vi "cCRDS Server.vi"(11 "cCRDS":refnum<class "cCRDS.lvclass">) -> ()   [LabVIEW 2015]
uses:
  cCRDS.lvclass
  Reusable/Instrument/state.ctl
  Reusable/CRDS/Main/CRDS.lvclass/CRDS.ctl
  Reusable/CRDS/Main/Read CRD RD Data Obs.vi
  Reusable/CRDS/Main/Write CRD RD Data Obs.vi
  Reusable/File IO/Class/File Observer.lvclass
  Reusable/Instrument/Instrument.lvclass
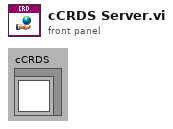
[diagram p1: front panel]
types:
  T1 = typedef "Instrument.lvclass/state.ctl" = enum8{"Configure", "Acquire", "Wait", "Quit", "Handle Error", "NOOP"}
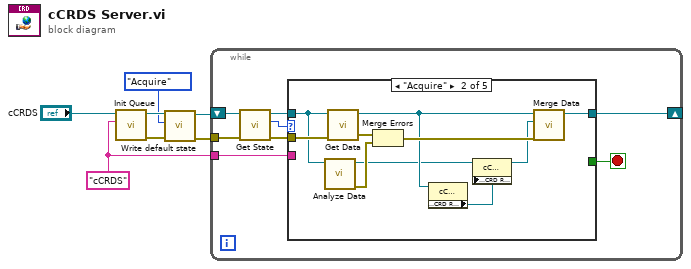
[diagram p0: block diagram]
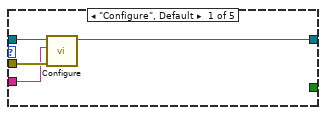
[diagram p2: hidden frame]
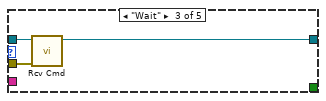
[diagram p3: hidden frame]
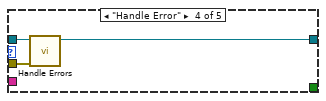
[diagram p4: hidden frame]
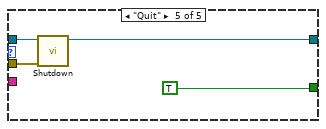
[diagram p5: hidden frame]
diagram:
  w4 = "cCRDS" ("queue_name")
  n1 = call "Init Queue.vi"("queue_name"=w4, "Instrument in"="cCRDS") -> ("error out"=w6:errorcluster, "Instrument out"=w7:refnum<class "cCRDS.lvclass">)  [unwired: 8 in]
  n2 = call "Write default state.vi"("error in (no error)"=w6, "instr state"=state."Acquire", "Instrument in"=w7) -> ("error out"=w1:errorcluster, "Instrument out"=w2:refnum<class "cCRDS.lvclass">)  [unwired: 7 in]
  n3 = while "Acquisition" {
    tunnel: w1 -> [w15]
    shift-right: [w8] -> _
    shift-left: w2 -> [w13]
    tunnel: w4 -> [w9]
    stop <- w10 stop-if-true
    n4 = call "Get State.vi"("error in"=w15, "Instrument in"=w13) -> ("error out"=w11:errorcluster, "default state"=w14:T1, "Instrument out"=w12:refnum<class "cCRDS.lvclass">)  [unwired: 7 in]
    n5 = case shown="\"Acquire\"" w14 {
      tunnel: w12 -> [w19 w24 w32 w35 w38]
      tunnel: w11 -> [w18 w29 w31 w34 w37]
      tunnel: [_ _ _ _ TRUE] -> w10
      tunnel: [w17 w26 w30 w33 w36] -> w8
      tunnel: w9 -> [w16 _ _ _ _]
      frame "Configure", Default {
        n6 = call-dynamic "Configure.vi"("error in"=w18, "name"=w16, "cCRDS in"=w19) -> ("cCRDS out"=w17:refnum<class "cCRDS.lvclass">)  [unwired: 7 in, 1 out]
      }
      frame "Acquire" {
        n7 = call-dynamic "Analyze Data.vi"("cCRDS in"=w24) -> ("error out"=w27:errorcluster, "cCRDS out"=w22:refnum<class "cCRDS.lvclass">)  [unwired: 9 in]
        n8 = call-dynamic "Get Data.vi"("error in"=w29, "cCRDS in"=w24) -> ("error out"=w28:errorcluster, "cCRDS_new out"=w23:refnum<class "cCRDS.lvclass">)  [unwired: 8 in]
        n9 = Merge Errors(w28, w27) -> (w25:errorcluster)
        n10 = property class="cCRDS"(reference=w23) -> ("Accessors:CRD RD Data Obs"=w20:refnum<class "File Observer.lvclass">)  [unwired: 1 in, 2 out]
        n11 = property class="cCRDS"(reference=w22, "Accessors:CRD RD Data Obs"=w20) -> (reference out=w21:refnum<class "cCRDS.lvclass">)  [unwired: 1 in, 1 out]
        n12 = call-dynamic "Merge Data.vi"("error in"=w25, "Analyzed"=w21, "Acquired"=w23) -> ("CRDS out"=w26:refnum<class "cCRDS.lvclass">)  [unwired: 7 in, 1 out]
      }
      frame "Wait" {
        n13 = call-dynamic "Rcv Cmd.vi"("error in"=w31, "cCRDS in"=w32) -> ("cCRDS out"=w30:refnum<class "cCRDS.lvclass">)  [unwired: 8 in, 1 out]
      }
      frame "Handle Error" {
        n14 = call-dynamic "Handle Errors.vi"("error in"=w34, "cCRDS_new in"=w35) -> ("cCRDS_new out"=w33:refnum<class "cCRDS.lvclass">)  [unwired: 7 in, 2 out]
      }
      frame "Quit" {
        n15 = call-dynamic "Shutdown.vi"("error in"=w37, "cCRDS_new in"=w38) -> ("cCRDS_new out"=w36:refnum<class "cCRDS.lvclass">)  [unwired: 8 in, 1 out]
      }
    }
  }
